vi "sampling_conditions.vi"() -> ()   [LabVIEW 2021]
panel:
  out "Sweep 2 Point Checker":string
  out "Sweep 2 Pot Check":string
  out "Sweep 1 Point Checker":string
  out "Sweep 1 Pot Check":string
  out "Gate Point number Checker":string
  out "Gate Potential_checker":string
  out "DorG_2":string
  out "DorG_1":string
  in  "VIntegration_2":dbl=100.0
  in  "VIntegration_1":dbl=100.0
  out "V Step_2 2":dbl
  out "V Step_1 2":dbl
  out "V Step_0 2":dbl
  out "V Step_2":dbl
  out "V Step_1":dbl
  out "V Step_0":dbl
  in  "Vvar_2_points":dbl
  in  "Vvar_1_points":dbl
  in  "Vvar_0_points":dbl
  in  "DorG_0":string(combo)
  in  "Vvar_2_Stop":dbl
  in  "Vvar_1_Stop":dbl
  in  "Vvar_0_Stop":dbl
  in  "Vvar_2_start":dbl
  in  "Vvar_1_start":dbl
  in  "Vvar_0_start":dbl
  in  "# Cycles":dbl
  in  "Sweep Spacing_2":string(combo)
  in  "Sweep Spacing_1":string(combo)
  in  "Sweep Spacing_0":string(combo)
  in  "VIntegration_0":dbl=100.0
  in  "Gate Current Compliance 2":dbl=1e-06
  in  "Gate Current Compliance 1":dbl=1e-06
  in  "Gate Current Compliance 0":dbl=1e-06
  in  "Drain Current Compliance 2":dbl=0.0001 format="%#_6p"
  in  "Drain Current Compliance 1":dbl=0.0001 format="%#_6p"
  in  "Drain Current Compliance":dbl=1e-06
  in  "Sweep 2":bool
  in  "Sweep 0":bool
  in  "Set Swe_2_Mode":string
  in  "Set Swe_1_Mode":string
  in  "Set Swe_0_Mode":string
  in  "Vvar-2_delaytime":dbl
  in  "Vvar-1_delaytime":dbl
  in  "Vvar-0_delaytime":dbl
  in  "Vvar_2_holdtime":dbl
  in  "Vvar_1_holdtime":dbl
  in  "Vvar_0_holdtime":dbl
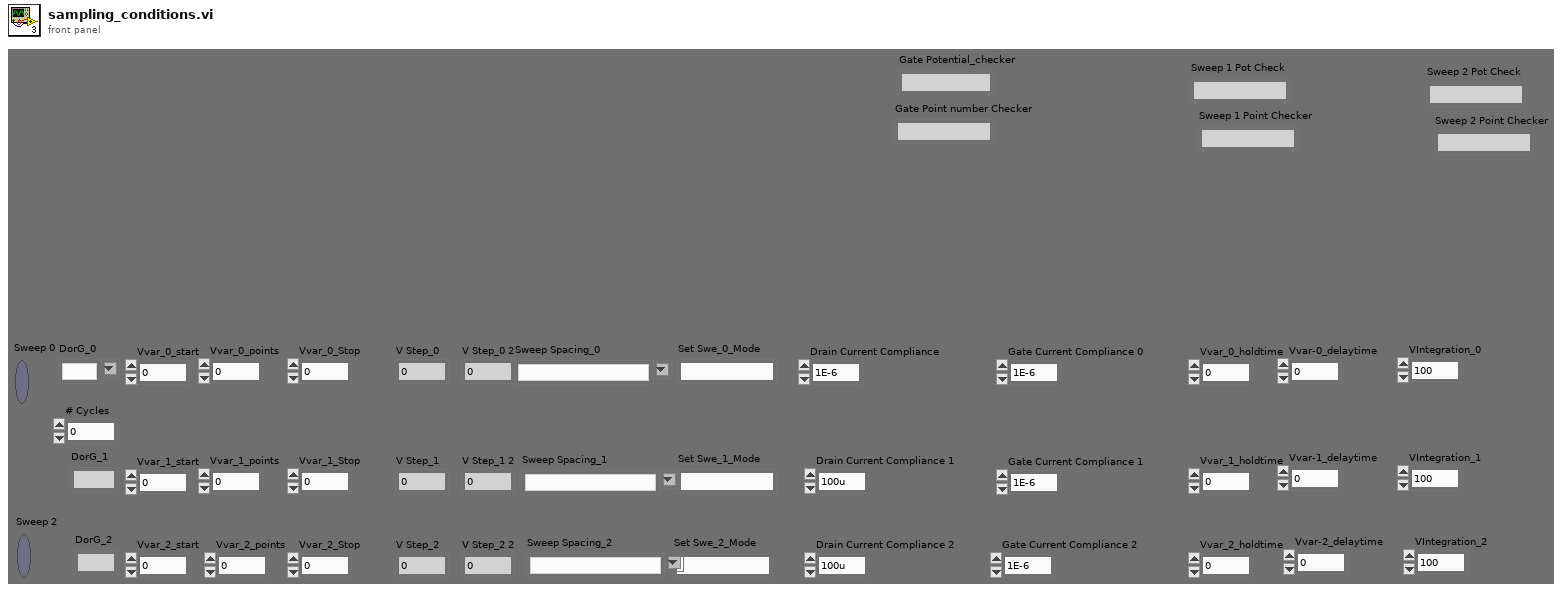
[diagram p1: front panel]
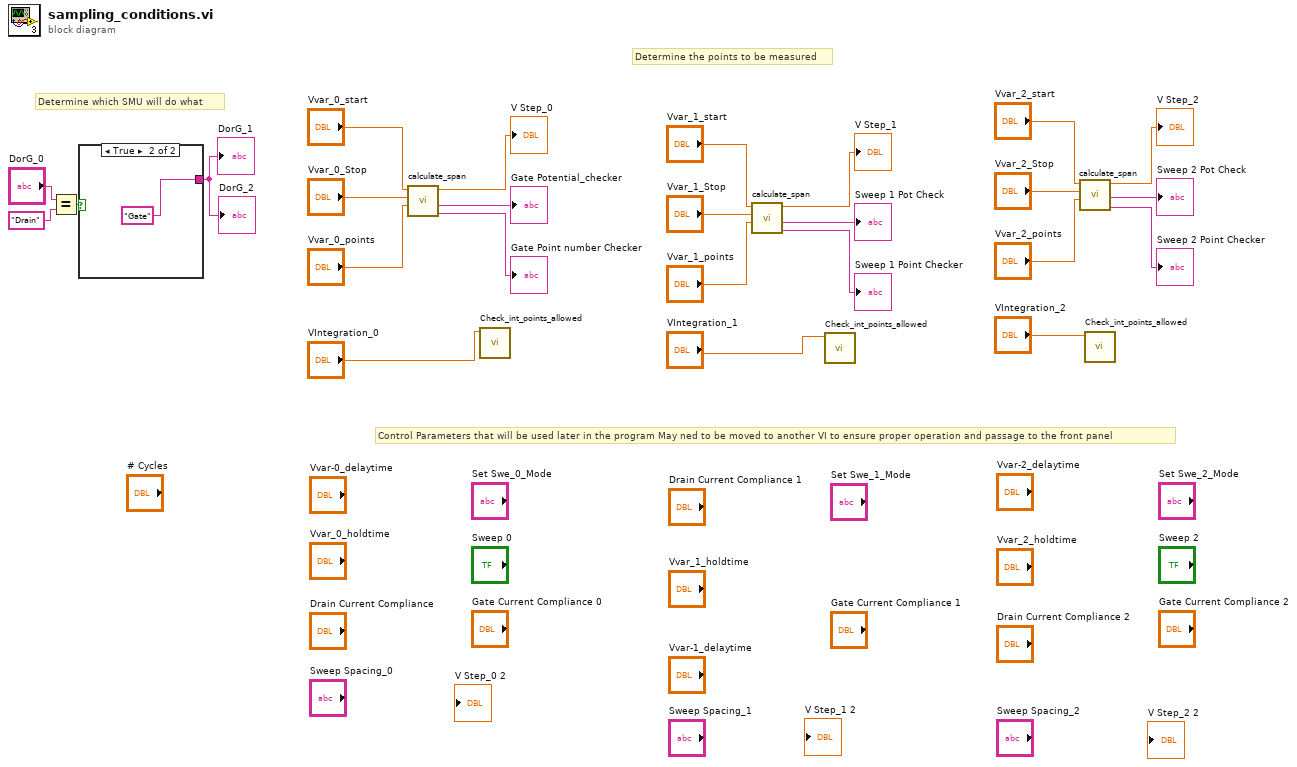
[diagram p0: block diagram]
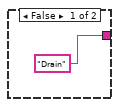
[diagram p2: hidden frame]
diagram:
  # "Control Parameters that will be used later in the program May ned to be moved to another VI to ensure proper operation and passage to the front panel"
  # "Determine which SMU will do what"
  # "Determine the points to be measured"
  n1 = Equal?(x="DorG_0", y="Drain") -> (x = y?=w20:bool)
  n2 = case shown="True" w20 {
    tunnel: ["Drain" "Gate"] -> w19
    frame False {
    }
    frame True {
    }
  }
  "DorG_1" <- w19
  "DorG_2" <- w19
  n3 = call "calculate_span.vi"("V_points"="Vvar_0_points", "V_Stop"="Vvar_0_Stop", "Vstart"="Vvar_0_start") -> ("Gate Point number Checker"=→"Gate Point number Checker":string, "Gate Potential_checker"=→"Gate Potential_checker":string, "V Step"=→"V Step_0":dbl)  [unwired: 6 in]
  n4 = call "Check_int_points_allowed.vi"("Integration Points"="VIntegration_0") -> ()  [unwired: 9 in, 2 out]
  n5 = call "calculate_span.vi"("V_points"="Vvar_1_points", "V_Stop"="Vvar_1_Stop", "Vstart"="Vvar_1_start") -> ("Gate Point number Checker"=→"Sweep 1 Point Checker":string, "Gate Potential_checker"=→"Sweep 1 Pot Check":string, "V Step"=→"V Step_1":dbl)  [unwired: 6 in]
  n6 = call "Check_int_points_allowed.vi"("Integration Points"="VIntegration_1") -> ()  [unwired: 9 in, 2 out]
  n7 = call "calculate_span.vi"("V_points"="Vvar_2_points", "V_Stop"="Vvar_2_Stop", "Vstart"="Vvar_2_start") -> ("Gate Point number Checker"=→"Sweep 2 Point Checker":string, "Gate Potential_checker"=→"Sweep 2 Pot Check":string, "V Step"=→"V Step_2":dbl)  [unwired: 6 in]
  n8 = call "Check_int_points_allowed.vi"("Integration Points"="VIntegration_2") -> ()  [unwired: 9 in, 2 out]
